vi "Read.vi"(8 "error in (no error)":errorcluster, 11 "Numeric in":refnum<class "Var_WFM.lvclass">) -> (0 "error out":errorcluster, 2 "Value":T1, 3 "Numeric out":refnum<class "Var_WFM.lvclass">)   [LabVIEW 2021, in "Var_WFM.lvclass"]
uses:
  Var_WFM.lvclass
  Type.ctl
  Var_WFM.lvclass/Var_WFM.ctl
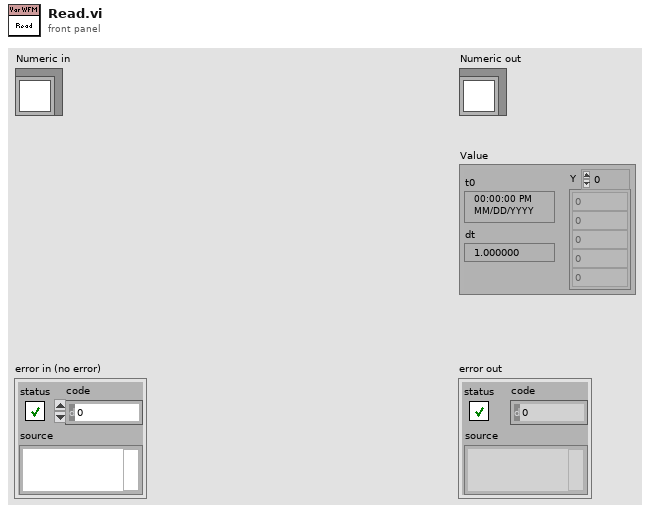
[diagram p1: front panel]
types:
  T1 = typedef "Var_WFM.lvclass/Type.ctl" = waveform(dbl)
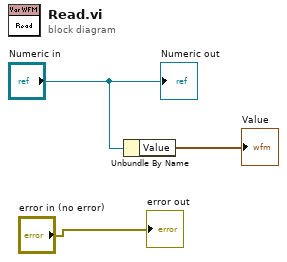
[diagram p0: block diagram]
diagram:
  n1 = Unbundle By Name("Numeric in") -> ("Value"=→"Value":T1)
  "error out" <- "error in (no error)"
  "Numeric out" <- "Numeric in"
